vi "I32 Image Data to PNG.vi"(8 "error in (no error)":errorcluster, 9 "Image Data":i32[][](array[numeric]), 10 "Image Name":string="INT Sum", 11 "Folder Path":path) -> (0 "error out":errorcluster, 3 "PNG File Path":path)   [LabVIEW 2021, in "Image.lvlib"]
uses:
  Image.lvlib
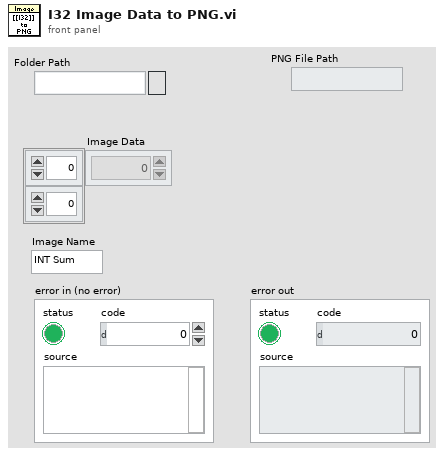
[diagram p1: front panel]
types:
  T1 = typedef "Image Type" = u32
  T2 = typedef "IMAQ Image.ctl" = refnum<image>
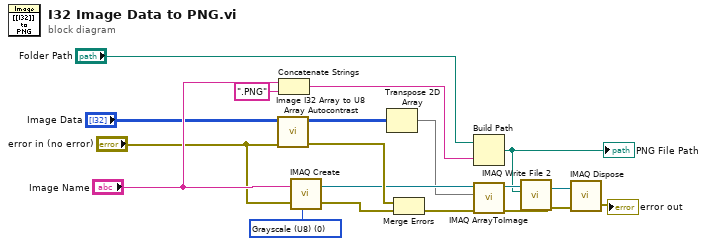
[diagram p0: block diagram]
diagram:
  w5 = T1 0 items=["Grayscale (U8)", "Grayscale (I16)", "Grayscale (SGL)", "Complex (CSG)", "RGB (U32)", "HSL (U32)", "RGB (U64)", "Grayscale (U16)"] ("Image Type")
  n1 = call "Image I32 Array to U8 Array Autocontrast.vi"("Error In"="error in (no error)", "I32 Image"="Image Data") -> ("Error Out"=w19:errorcluster, "U8 5-95% Contrast Enhanced U8 Image"=w17:u8[][])  [unwired: 8 in]
  n2 = Concatenate Strings("Image Name", ".PNG" ("string")) -> (w9:string)
  n3 = call "IMAQ Create"("Image Name"="Image Name", "Image Type"=w5, "error in (no error)"="error in (no error)") -> ("New Image"=w11:T2, "error out"=w12:errorcluster)  [unwired: 2 in]
  n4 = Transpose 2D Array(2D array=w17) -> (transposed array=w7:u8[][])
  n5 = Merge Errors(w19, w12) -> (w18:errorcluster)
  n6 = Build Path(base path="Folder Path", name or relative path=w9) -> (appended path=w10:path)
  "PNG File Path" <- w10
  n7 = call "IMAQ ArrayToImage"("error in (no error)"=w18, "Image Pixels (U8)"=w7, "Image"=w11) -> ("error out"=w16:errorcluster, "Image Out"=w14:T2)  [unwired: 7 in]
  n8 = call-poly "IMAQ Write File 2"("error in (no error)"=w16, "File Path"=w10, "Image"=w14) -> ("error out"=w3:errorcluster, "Image Out (duplicate)"=w2:T2)  [unwired: 7 in]
  n9 = call "IMAQ Dispose"("Image"=w2, "error in (no error)"=w3) -> ("error out"=→"error out":errorcluster)  [unwired: 4 in]
